vi "GetType.vi"(8 "error in (no error)":errorcluster, 11 "Read Multi-Point [MP] Msg":refnum<class "Read Multi-Point [MP] Msg.lvclass">) -> (0 "error out":errorcluster, 2 "Data Sample":variant, 3 "Read Multi-Point [MP] Msg":refnum<class "Read Multi-Point [MP] Msg.lvclass">)   [LabVIEW 2016, in "CS++DMM.lvlib" / "Read Multi-Point [MP] Msg.lvclass"]
uses:
  Read Multi-Point [MP] Msg.lvclass
  Read Multi-Point [MP] Msg.lvclass/Read Multi-Point [MP] Msg.ctl
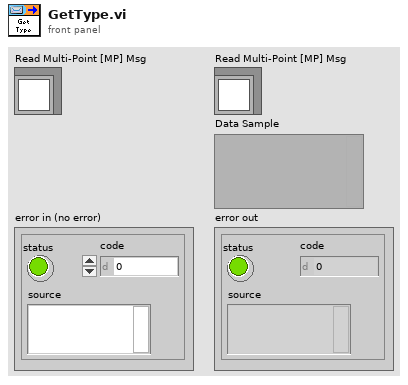
[diagram p1: front panel]
types:
  T1 = cluster{"maximum time (5s)":dbl[unit], "array size":i32}
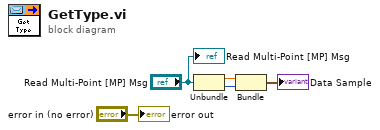
[diagram p0: block diagram]
diagram:
  n1 = Unbundle("Read Multi-Point [MP] Msg") -> (w2:dbl[unit], w1:i32)
  n2 = Bundle("maximum time (5s)"=w2, "array size"=w1) -> (→"Data Sample":T1)  [unwired: 1 in]
  "error out" <- "error in (no error)"
  "Read Multi-Point [MP] Msg" <- "Read Multi-Point [MP] Msg"
